vi "BoolText AsUnicode.vi"(0 "Ctl Refnum":refnum<vi>, 5 "Caption.Interpret As Unicode":bool, 11 "error in":errorcluster) -> (4 "reference out":refnum<vi>, 15 "error out":errorcluster)   [LabVIEW 2017]
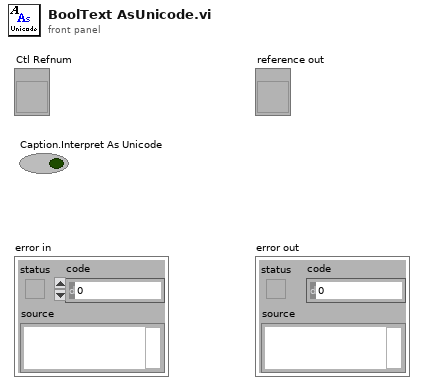
[diagram p1: front panel]
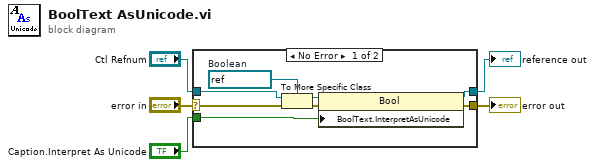
[diagram p0: block diagram]
diagram:
  n1 = case shown="No Error" "error in" {
    selector: "error in" -> [w10 w14]
    tunnel: "Ctl Refnum" -> [w9 w15]
    tunnel: "Caption.Interpret As Unicode" -> [w13 _]
    tunnel: [w12 w14] -> w3
    tunnel: [w11 w15] -> w2
    frame No Error {
      w8 = refnum<vi> refnum  # Boolean
      n2 = To More Specific Class(target class=w8, reference=w9, error in=w10) -> (specific class reference=w7:refnum<vi>, error out=w6:errorcluster)
      n3 = property class="Bool"(reference=w7, error in=w6, "BoolText.InterpretAsUnicode"=w13) -> (reference out=w11:refnum<vi>, error out=w12:errorcluster)
    }
    frame Error {
    }
  }
  "error out" <- w3
  "reference out" <- w2
